vi "Create Channel Task Manual.vi"(8 "error in (no error)":errorcluster, 10 "Data":T1[](array[typedef]), 11 "PWM Output in":refnum<class "PWM Output.lvclass">) -> (0 "error out":errorcluster, 3 "PWM Output out":refnum<class "PWM Output.lvclass">)   [LabVIEW 2023, in "HardwareAbstractionLayer_LVOOP.lvlib" / "PWM Output.lvclass"]
uses:
  PWM Output.lvclass
  GUI/Actor/Diagnostic/Instruments UI/PWM Output/Control/PWM Output.ctl
  GUI/Actor/Diagnostic/Diagnostic.lvlib
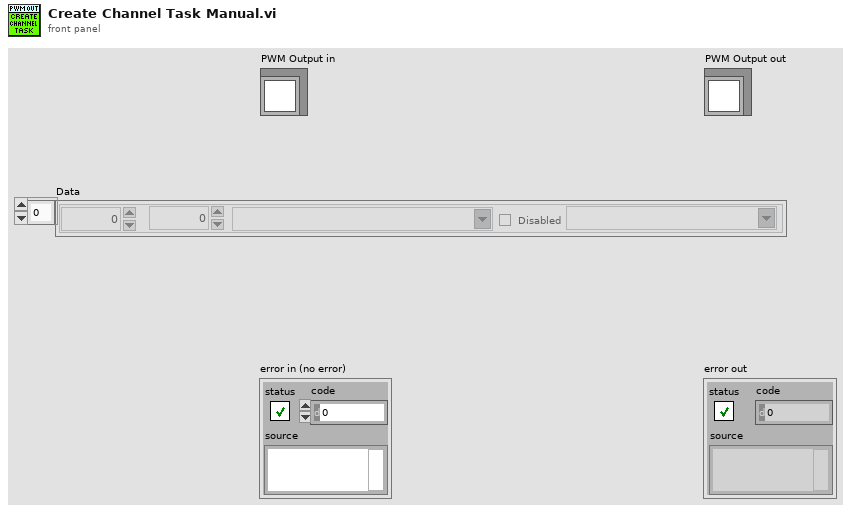
[diagram p1: front panel]
types:
  T1 = typedef "GUI.lvlib/Diagnostic.lvlib/PWM Output.ctl" = cluster{"Frequency":dbl, "Duty Cycles":dbl, "Terminal":tag, "Enable":bool, "Physical Channel":tag}
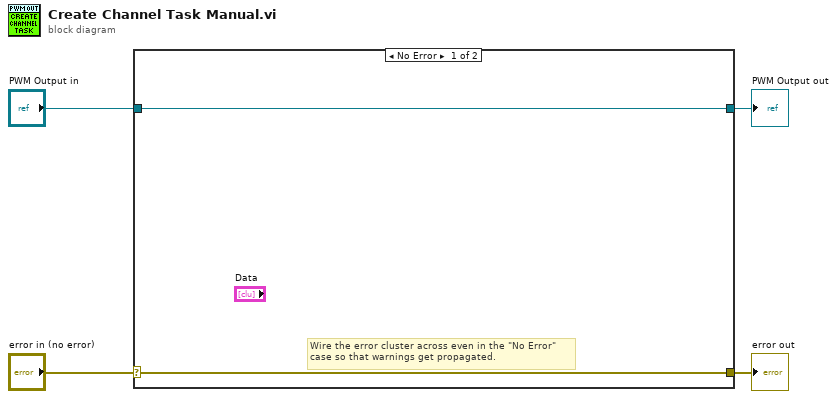
[diagram p0: block diagram]
diagram:
  n1 = case shown="No Error" "error in (no error)" {
    selector: "error in (no error)" -> [w5 w8]
    tunnel: [w5 w8] -> w3
    tunnel: [w6 w7] -> w1
    tunnel: "PWM Output in" -> [w6 w7]
    frame No Error {
      # "Wire the error cluster across even in the \"No Error\"\ncase so that warnings get propagated."
    }
    frame Error {
    }
  }
  "error out" <- w3
  "PWM Output out" <- w1
